vi "3BLABVIEW.vi"() -> ()   [LabVIEW 2013]
panel:
  out "min index(es)":i32
  out "min value":dbl
  out "max index(es)":i32
  out "max value":dbl
  in  "Array":dbl[](array[numeric])
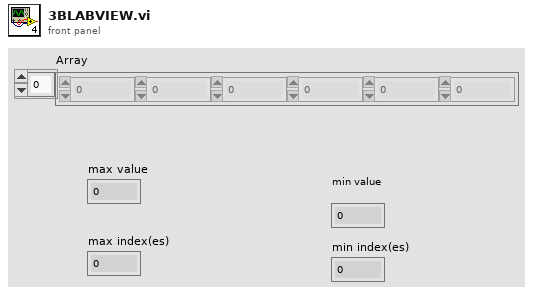
[diagram p1: front panel]
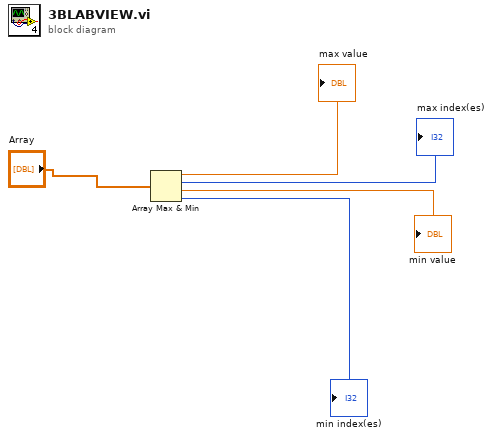
[diagram p0: block diagram]
diagram:
  n1 = Array Max & Min(array="Array") -> (max value=→"max value":dbl, max index (indices)=→"max index(es)":i32, min value=→"min value":dbl, min index (indices)=→"min index(es)":i32)
